vi "NephGFV.vi"(8 "error in (no error)":errorcluster, 10 "NephDataEnum":T1, 11 "Variant In":variant) -> (0 "error out":errorcluster, 3 "Variant Out":variant)   [LabVIEW 2013]
doc: "Use this template to build a VI to use as a subVI."
uses:
  NephDataEnum.ctl
  NephDataCluster.ctl
panel:
  in  "Array":dbl[](array[numeric])
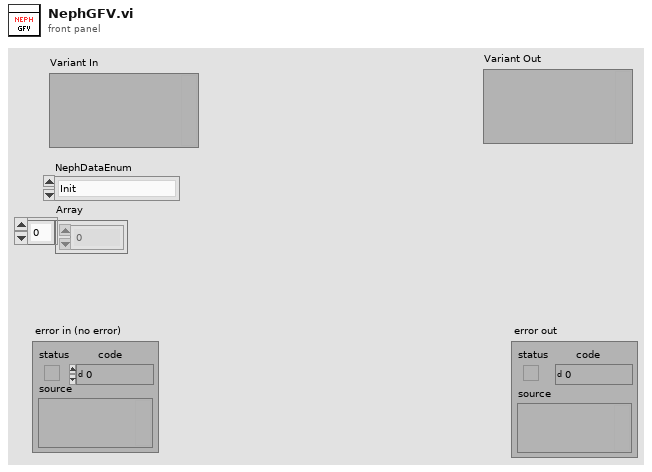
[diagram p1: front panel]
types:
  T1 = typedef "NephDataEnum.ctl" = enum16{"Init", "Insert Measurement", "Read Buffer Size", "Write Buffer Size", "Read Current Measurement", "Read Buffered Meas"}
  T2 = cluster{"Duration(counts)":i32, "NumberOfDataPoints":i32}
  T3 = typedef "NephDataCluster.ctl" = cluster{"dateTime":string, "unitNo":string, "RF_PMT":dbl, "RF_REF":dbl, "GF_PMT":dbl, "GF_REF":dbl, "BF_PMT":dbl, "BF_REF":dbl, "RB_PMT":dbl, "RB_REF":dbl, "GB_PMT":dbl, "GB_REF":dbl, "BB_PMT":dbl, "BB_REF":dbl, "Temp":dbl, "Pressure":dbl, "RH":dbl, "PMT_DARK":dbl, "Forw_Dark_Ref":dbl, "Back_Dark_Ref":dbl, "Back_Scatt_Red":dbl, "Back_Scatt_Green":dbl, "Back_Scatt_Blue":dbl, "Total_Scatt_Red":dbl, "Total_Scatt_Green":dbl, "Total_Scatt_Blue":dbl, "Fan_RPM":dbl, "AngstromRG":dbl, "AngstromRB":dbl, "AngstromBG":dbl, "BackTotalRatioRed":dbl, "BackTotalRatioGreen":dbl, "BackTotalRatioBlue":dbl}
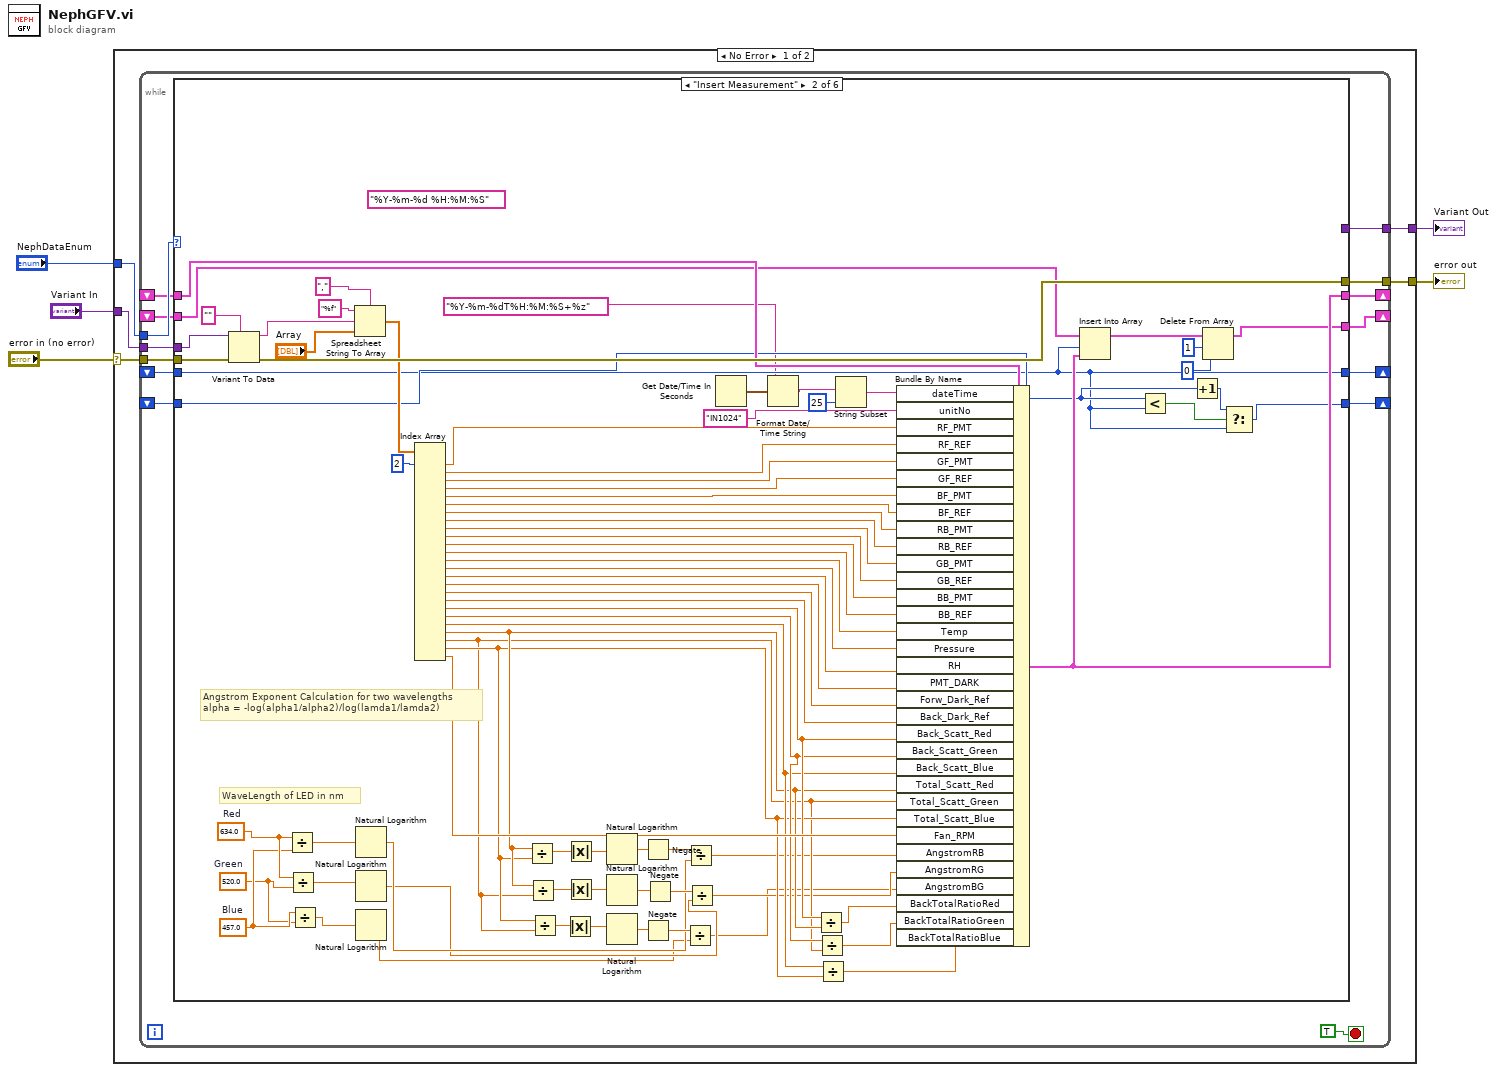
[diagram p0: block diagram]
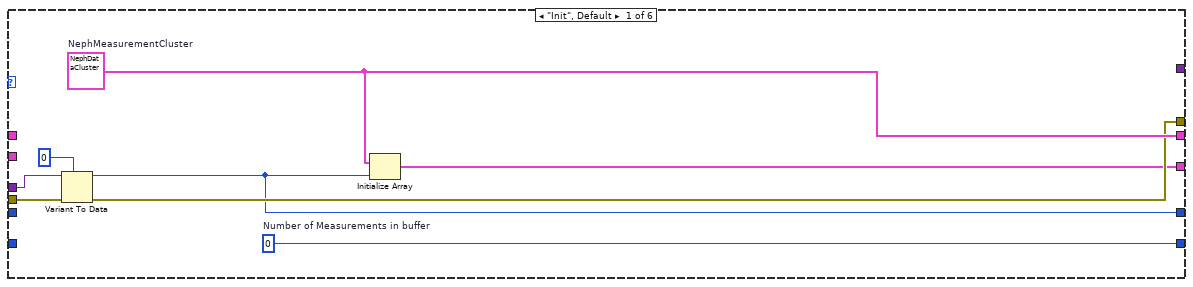
[diagram p2: hidden frame]
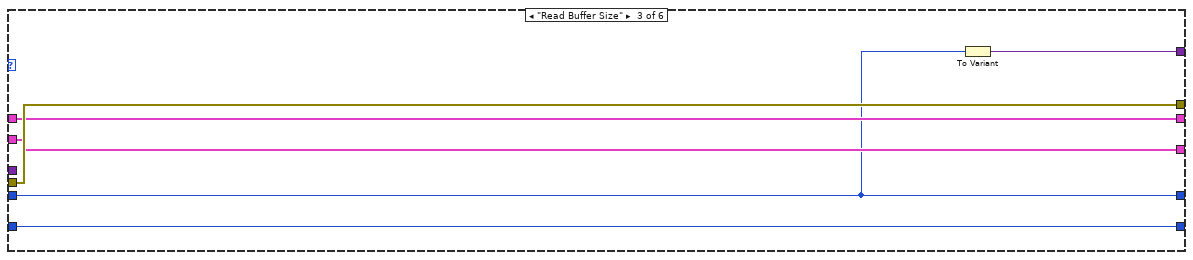
[diagram p3: hidden frame]
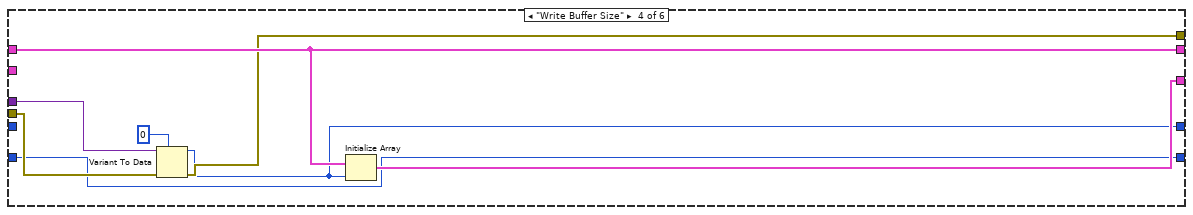
[diagram p4: hidden frame]
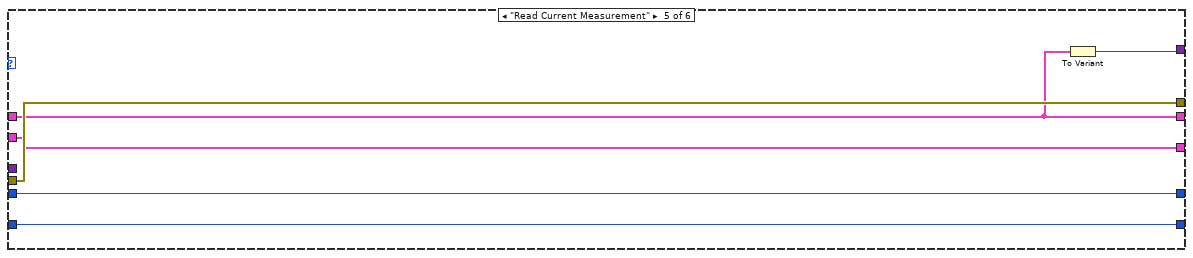
[diagram p5: hidden frame]
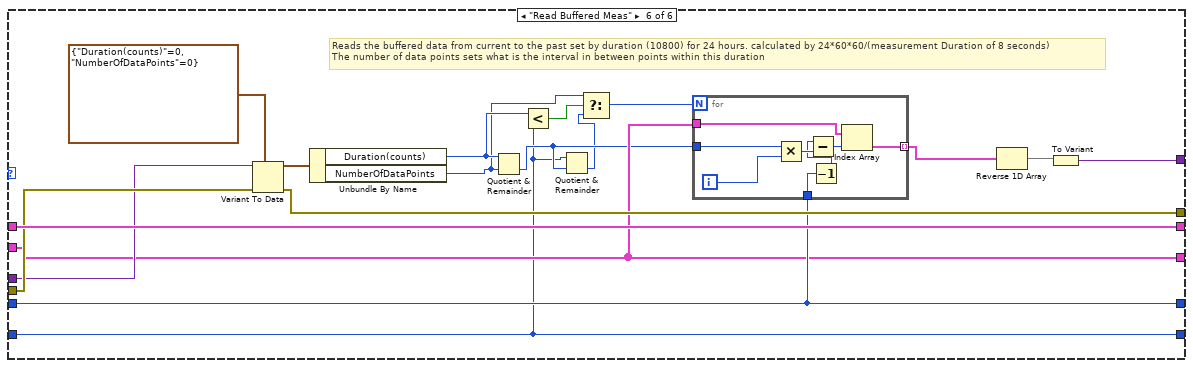
[diagram p6: hidden frame]
diagram:
  n1 = case shown="No Error" "error in (no error)" {
    selector: "error in (no error)" -> [w8 w159]
    tunnel: [w7 w159] -> w4
    tunnel: "NephDataEnum" -> [w10 _]
    tunnel: "Variant In" -> [w9 _]
    tunnel: [w6 _] -> w1
    frame No Error {
      n2 = while {
        tunnel: w10 -> [w23]
        shift-right: [w22] -> _
        shift-left: _ -> [w17]
        tunnel: w9 -> [w21]
        tunnel: w8 -> [w20]
        tunnel: [w19] -> w7
        shift-right: [w18] -> _
        shift-left: _ -> [w16]
        shift-right: [w15] -> _
        shift-left: _ -> [w14]
        tunnel: [w13] -> w6
        shift-right: [w12] -> _
        shift-left: _ -> [w11]
        stop <- TRUE stop-if-true
        n3 = case shown="\"Insert Measurement\"" w23 {
          tunnel: [w32 w81 w117 w124 w128 w150] -> w22
          tunnel: w21 -> [w31 w112 _ w126 _ w146]
          tunnel: w20 -> [w30 w111 w118 w122 w132 w147]
          tunnel: [w28 w109 w118 w121 w132 w145] -> w19
          tunnel: [w27 w77 w116 w123 w131 w142] -> w18
          tunnel: w17 -> [_ w102 w117 w124 w128 w150]
          tunnel: w16 -> [_ w82 w116 _ w131 w142]
          tunnel: [w26 w70 w114 w120 w130 w143] -> w15
          tunnel: w14 -> [_ w70 w114 _ w130 w143]
          tunnel: [_ _ w115 _ w129 w149] -> w13
          tunnel: [w25 w71 w113 w119 w127 w136] -> w12
          tunnel: w11 -> [_ w73 w113 w119 w127 w136]
          frame "Init", Default {
            w25 = 0  # Number of Measurements in buffer
            w32 = T3 {"dateTime"="", "unitNo"="", "RF_PMT"=0.0, "RF_REF"=0.0, "GF_PMT"=0.0, "GF_REF"=0.0, "BF_PMT"=0.0, "BF_REF"=0.0, "RB_PMT"=0.0, "RB_REF"=0.0, "GB_PMT"=0.0, "GB_REF"=0.0, "BB_PMT"=0.0, "BB_REF"=0.0, "Temp"=0.0, "Pressure"=0.0, "RH"=0.0, "PMT_DARK"=0.0, "Forw_Dark_Ref"=0.0, "Back_Dark_Ref"=0.0, "Back_Scatt_Red"=0.0, "Back_Scatt_Green"=0.0, "Back_Scatt_Blue"=0.0, "Total_Scatt_Red"=0.0, "Total_Scatt_Green"=0.0, "Total_Scatt_Blue"=0.0, "Fan_RPM"=0.0, "AngstromRG"=0.0, "AngstromRB"=0.0, "AngstromBG"=0.0, "BackTotalRatioRed"=0.0, "BackTotalRatioGreen"=0.0, "BackTotalRatioBlue"=0.0}  # NephMeasurementCluster
            n4 = Variant To Data(error in=w30, type=0, Variant=w31) -> (data=w26:i32, error out=w28:errorcluster)
            n5 = Initialize Array(w32, w26) -> (w27:T3[])
          }
          frame "Insert Measurement" {
            w62 = 457.0  # Blue
            w61 = 520.0  # Green
            w63 = 634.0  # Red
            (unwired) "%Y-%m-%d %H:%M:%S" ("time format string (%c)")
            # "Angstrom Exponent Calculation for two wavelengths\nalpha = -log(alpha1/alpha2)/log(lamda1/lamda2)"
            # "WaveLength of LED in nm"
            n6 = Variant To Data(error in=w111, type="", Variant=w112) -> (data=w105:string, error out=w109:errorcluster)
            n7 = Divide(x=w63, y=w62) -> (x/y=w60:dbl)
            n8 = Divide(x=w63, y=w61) -> (x/y=w58:dbl)
            n9 = Divide(x=w62, y=w61) -> (x/y=w59:dbl)
            n10 = Spreadsheet String To Array(delimiter (Tab)=",", format string="%f", spreadsheet string=w105, array type (2D Dbl)="Array") -> (array=w104:dbl[])
            n11 = Natural Logarithm(1:w60) -> (0:w48:dbl)
            n12 = Natural Logarithm(1:w58) -> (0:w47:dbl)
            n13 = Natural Logarithm(1:w59) -> (0:w46:dbl)
            n14 = Index Array(array=w104, index #1=2 ("index")) -> (element #1=w101:dbl, element #2=w100:dbl, element #3=w99:dbl, element #4=w98:dbl, element #5=w97:dbl, element #6=w96:dbl, element #7=w95:dbl, element #8=w94:dbl, element #9=w93:dbl, element #10=w92:dbl, element #11=w91:dbl, element #12=w90:dbl, element #13=w89:dbl, element #14=w88:dbl, element #15=w87:dbl, element #16=w86:dbl, element #17=w85:dbl, element #18=w84:dbl, element #19=w69:dbl, element #20=w68:dbl, element #21=w67:dbl, element #22=w57:dbl, element #23=w55:dbl, element #24=w56:dbl, element #25=w83:dbl)  [unwired: 24 in]
            n15 = Divide(x=w57, y=w56) -> (x/y=w38:dbl)
            n16 = Divide(x=w57, y=w55) -> (x/y=w39:dbl)
            n17 = Divide(x=w56, y=w55) -> (x/y=w41:dbl)
            n18 = Absolute Value(x=w41) -> (abs(x)=w40:dbl)
            n19 = Absolute Value(x=w38) -> (abs(x)=w37:dbl)
            n20 = Absolute Value(x=w39) -> (abs(x)=w42:dbl)
            n21 = Natural Logarithm(1:w37) -> (0:w54:dbl)
            n22 = Natural Logarithm(1:w42) -> (0:w52:dbl)
            n23 = Natural Logarithm(1:w40) -> (0:w53:dbl)
            n24 = Negate(x=w54) -> (-x=w49:dbl)
            n25 = Negate(x=w53) -> (-x=w50:dbl)
            n26 = Negate(x=w52) -> (-x=w51:dbl)
            n27 = Divide(x=w50, y=w46) -> (x/y=w43:dbl)
            n28 = Divide(x=w49, y=w48) -> (x/y=w45:dbl)
            n29 = Divide(x=w51, y=w47) -> (x/y=w44:dbl)
            n30 = Get Date/Time In Seconds() -> (seconds since 1Jan1904=w75:timestamp)
            n31 = Format Date/Time String(time format string (%c)="%Y-%m-%dT%H:%M:%S+%z", seconds (now)=w75) -> (date/time string=w33:string)  [unwired: 1 in]
            n32 = Divide(x=w69, y=w57) -> (x/y=w66:dbl)
            n33 = Divide(x=w68, y=w55) -> (x/y=w65:dbl)
            n34 = Divide(x=w67, y=w56) -> (x/y=w64:dbl)
            n35 = String Subset(string=w33, length (rest)=25 ("length (rest)")) -> (substring=w34:string)  [unwired: 1 in]
            n36 = Bundle By Name(cluster=w102, "dateTime"=w34, "unitNo"="IN1024" ("UnitNumber"), "RF_PMT"=w101, "RF_REF"=w100, "GF_PMT"=w99, "GF_REF"=w98, "BF_PMT"=w97, "BF_REF"=w96, "RB_PMT"=w95, "RB_REF"=w94, "GB_PMT"=w93, "GB_REF"=w92, "BB_PMT"=w91, "BB_REF"=w90, "Temp"=w89, "Pressure"=w88, "RH"=w87, "PMT_DARK"=w86, "Forw_Dark_Ref"=w85, "Back_Dark_Ref"=w84, "Back_Scatt_Red"=w69, "Back_Scatt_Green"=w68, "Back_Scatt_Blue"=w67, "Total_Scatt_Red"=w57, "Total_Scatt_Green"=w55, "Total_Scatt_Blue"=w56, "Fan_RPM"=w83, "AngstromRB"=w45, "AngstromRG"=w44, "AngstromBG"=w43, "BackTotalRatioRed"=w66, "BackTotalRatioGreen"=w65, "BackTotalRatioBlue"=w64) -> (w81:T3)
            n37 = Insert Into Array "Insert Into Array"(array=w82, index=w70, new element=w81) -> (w80:T3[])
            n38 = Less?(x=w73, y=w70) -> (x < y?=w74:bool)
            n39 = Increment(x=w73) -> (x+1=w72:i32)
            n40 = Delete From Array "Delete From Array"(array=w80, length=1, index=0) -> (array with subset deleted=w77:T3[])  [unwired: 1 out]
            n41 = Select(t=w72, s=w74, f=w70) -> (s? t:f=w71:i32)
          }
          frame "Read Buffer Size" {
            n42 = To Variant(anything=w114) -> (Variant=w115:variant)
          }
          frame "Write Buffer Size" {
            n43 = Variant To Data(error in=w122, type=0, Variant=w126) -> (data=w120:i32, error out=w121:errorcluster)
            n44 = Initialize Array(w124, w120) -> (w123:T3[])
          }
          frame "Read Current Measurement" {
            n45 = To Variant(anything=w128) -> (Variant=w129:variant)
          }
          frame "Read Buffered Meas" {
            # "Reads the buffered data from current to the past set by duration (10800) for 24 hours. calculated by 24*60*60/(measurement Duration of 8 seconds)\nThe number of data points sets what is the interval in between points within this duration"
            n46 = Variant To Data(error in=w147, type=T2 {"Duration(counts)"=0, "NumberOfDataPoints"=0}, Variant=w146) -> (data=w144:T2, error out=w145:errorcluster)
            n47 = Unbundle By Name(w144) -> ("Duration(counts)"=w141:i32, "NumberOfDataPoints"=w139:i32)
            n48 = Quotient & Remainder(x=w141, y=w139) -> (floor(x/y)=w137:i32)  [unwired: 1 out]
            n49 = Less?(x=w141, y=w136) -> (x < y?=w140:bool)
            n50 = Quotient & Remainder(x=w136, y=w137) -> (floor(x/y)=w135:i32)  [unwired: 1 out]
            n51 = Select(t=w139, s=w140, f=w135) -> (s? t:f=w138:i32)
            n52 = for {
              N: w138 -> [_]
              tunnel: w143 -> [w153]
              tunnel: w142 -> [w155]
              tunnel: [w154] -> w134 mode=indexing
              tunnel: w137 -> [w151]
              i -> [w158]
              n53 = Multiply(x=w151, y=w158) -> (x*y=w156:i32)
              n54 = Decrement(x=w153) -> (x-1=w152:i32)
              n55 = Subtract(x=w152, y=w156) -> (x-y=w157:i32)
              n56 = Index Array(array=w155, index=w157) -> (element=w154:T3)
            }
            n57 = Reverse 1D Array(array=w134) -> (reversed array=w133:T3[])
            n58 = To Variant(anything=w133) -> (Variant=w149:variant)
          }
        }
      }
    }
    frame Error {
    }
  }
  "error out" <- w4
  "Variant Out" <- w1
